vi "to_json.vi"(8 "error in":errorcluster, 11 "target.video in":refnum<class "target.video.lvclass">) -> (0 "error out":errorcluster, 2 "json":string, 3 "target.video out":refnum<class "target.video.lvclass">, 4 "Not Default":bool)   [LabVIEW 2020, in "datasources.lvlib" / "target.video.lvclass"]
uses:
  target.video.lvclass
  C:/code/labview-client/lv_src/Nominal Client/datasources/target/target.lvclass
  target.video.lvclass/target.video.ctl
  target/target.lvclass/target.ctl
  dataset/dataset.lvclass/dataset.ctl
  428e81a4-e553-4bd8-9727-470612eb2722.vi
  44014f50-ab4e-42bf-98e0-f8910821d057.vi
  6f4a9cd9-95da-4d00-8da6-4a49d3ace755.vi
  b2da3fc4-5a27-4170-9632-6c616410d1ce.vi
  a8577a1a-19ab-4315-acfd-5959197f0bba.vi
  b13016ed-5689-47b0-9406-ea70241d4c20.vi
  dd574b23-1e1f-49d0-b409-8656717e9e11.vi
  target/properties.get.vi
  target/labels.get.vi
  target/dataset.get.vi
  target/channelConfig.get.vi
  target/workspace.get.vi
  dataset/datasetName.get.vi
  dataset/datasetDescription.get.vi
  dataset/rid.get.vi
  <vilib>/JDP Science/JSONtext/Variant to JSON Text.vi
  <vilib>/JDP Science/JSONtext/support/Format JSON Object.vi
  nominal types/properties/properties.lvclass
  nominal types/labels/labels.lvclass
  <vilib>/JDP Science/JSONtext/LVClass Serializer/JSONtext LVClass Serializer.lvclass
  dataset/dataset.lvclass
  nominal types/channelConfig/channelConfig.lvclass
  nominal types/workspace/workspace.lvclass
  <vilib>/JDP Science/JSONtext/JSONtext.lvlib
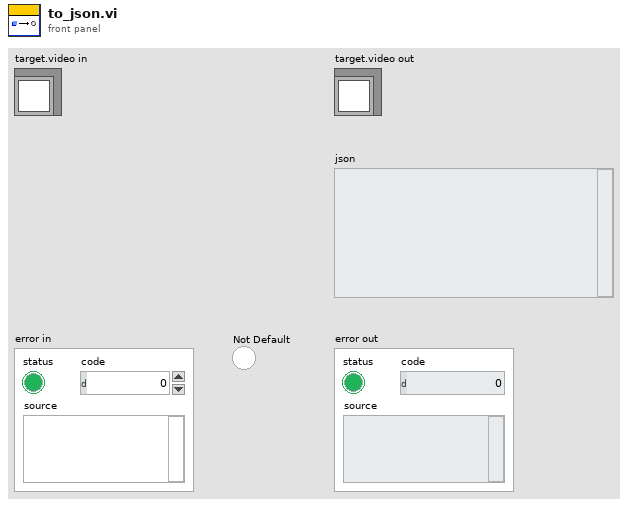
[diagram p1: front panel]
types:
  T1 = cluster{"type":string, "existing":cluster{"videoRid":string}}
  T2 = cluster{"Accessors:datasetName":string, "Accessors:datasetDescription":string}
  T3 = cluster{"Accessors:datasetName":bool, "Accessors:datasetDescription":bool}
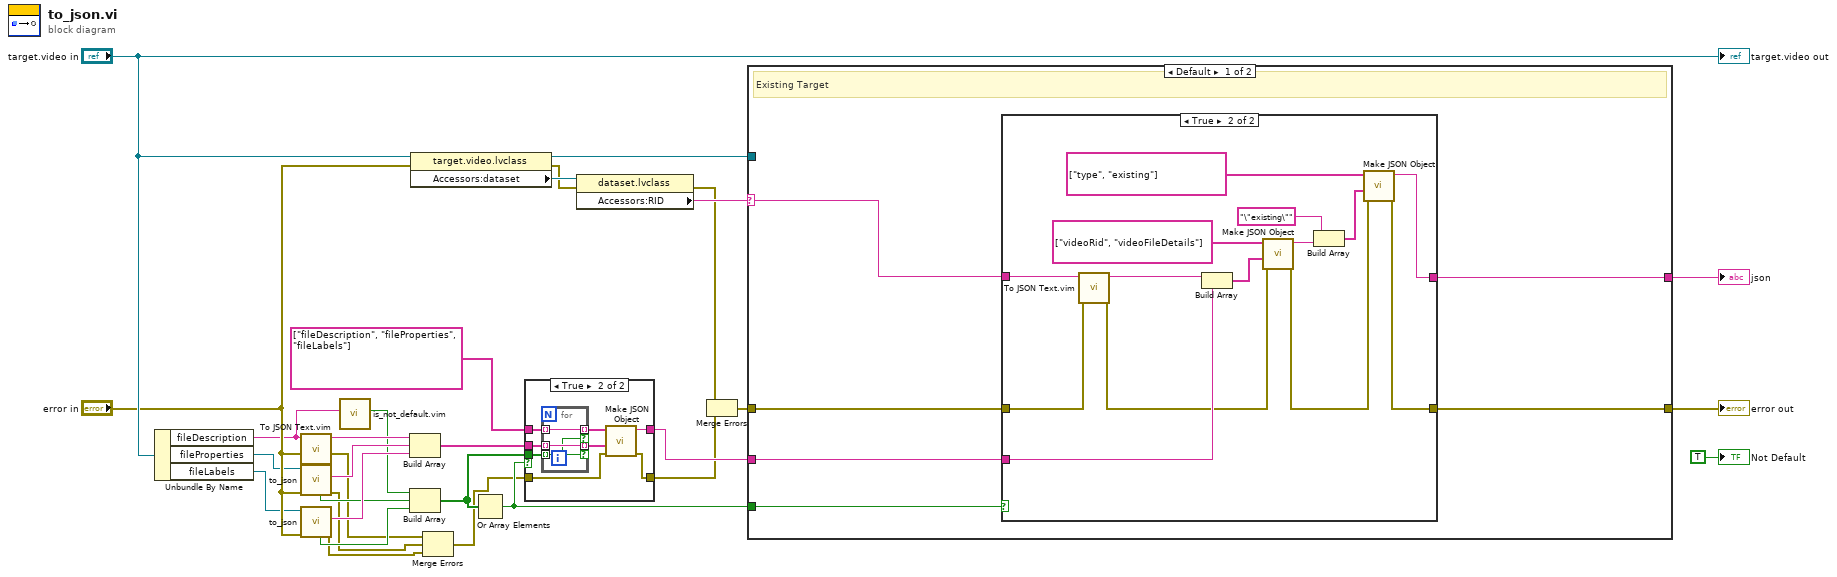
[diagram p0: block diagram]
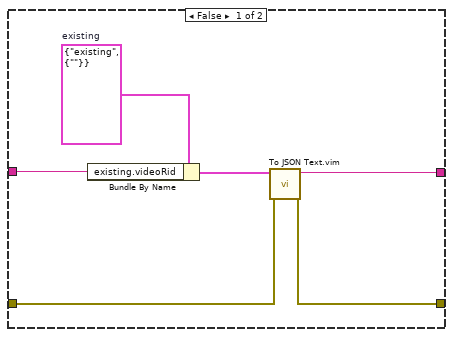
[diagram p3: hidden frame]
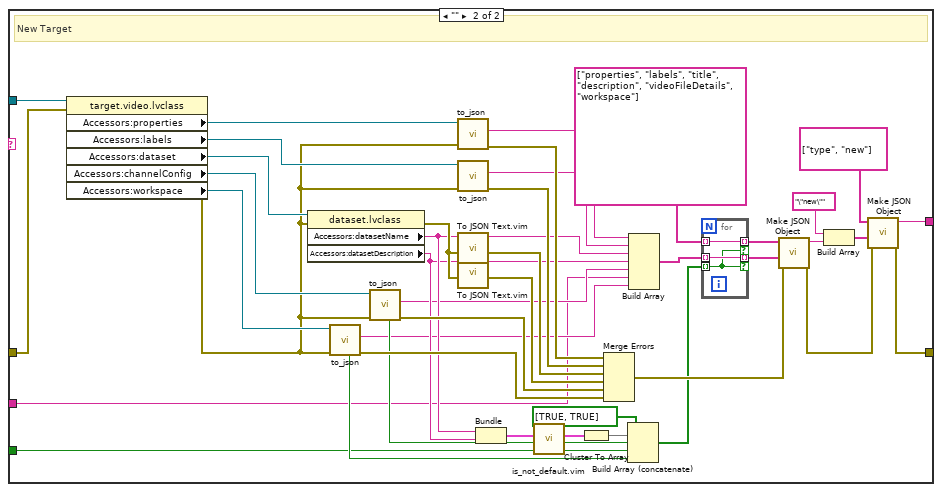
[diagram p4: hidden frame]
diagram:
  n1 = Unbundle By Name("target.video in") -> ("fileDescription"=w3:string, "fileProperties"=w2:refnum<class "properties.lvclass">, "fileLabels"=w1:refnum<class "labels.lvclass">)
  n2 = call "To JSON Text.vim"("error in (no error)"="error in", "Anything"=w3) -> ("error out"=w10:errorcluster, "<JSON>"=w20:string)  [unwired: 8 in]
  n3 = call-dynamic "to_json.vi"("error in"="error in", "properties in"=w2) -> ("error out"=w9:errorcluster, "json"=w22:string, "Not Default"=w18:bool)  [unwired: 6 in, 1 out]
  n4 = call-dynamic "to_json.vi"("error in"="error in", "labels in"=w1) -> ("error out"=w8:errorcluster, "json"=w21:string, "Not Default"=w19:bool)  [unwired: 6 in, 1 out]
  n5 = call "is_not_default.vim"("data"=w3) -> ("Not Default"=w17:bool)  [unwired: 10 in]
  n6 = Build Array(w20, w22, w21) -> (w23:string[])
  n7 = Build Array(w17, w18, w19) -> (w25:bool[])
  n8 = property class="target.video.lvclass"(reference="target.video in", error in="error in") -> (reference out=w13:refnum<class "target.video.lvclass">, error out=w11:errorcluster, "Accessors:dataset"=w29:refnum<class "dataset.lvclass">)
  n9 = Merge Errors(w10, w9, w8) -> (w7:errorcluster)
  n10 = Or Array Elements(Boolean array=w25) -> (logical OR=w14:bool)
  n11 = case shown="True" w14 {
    tunnel: w23 -> [_ w39]
    tunnel: string[] ["fileDescription", "fileProperties", "fileLabels"] ("Item Names") -> [_ w38]
    tunnel: w25 -> [_ w35]
    tunnel: [_ w34] -> w15
    tunnel: [w31 w33] -> w5
    tunnel: w7 -> [w31 w32]
    frame False {
    }
    frame True {
      n12 = for {
        tunnel: w39 -> [w42] mode=indexing
        tunnel: [w42] -> w36 mode=indexing if=w40
        tunnel: w38 -> [w41] mode=indexing
        tunnel: [w41] -> w37 mode=indexing if=w40
        tunnel: w35 -> [w40] mode=indexing
      }
      n13 = call <vilib>:"Make JSON Object.vi"("error in (no error)"=w32, "JSON Items"=w36, "Item Names"=w37) -> ("error out"=w33:errorcluster, "<JSON>"=w34:string)  [unwired: 7 in]
    }
  }
  n14 = property class="dataset.lvclass"(reference=w29, error in=w11) -> (error out=w6:errorcluster, "Accessors:RID"=w30:string)  [unwired: 1 out]
  n15 = Merge Errors(w6, w5) -> (w4:errorcluster)
  n16 = case shown="Default" w30 {
    selector: w30 -> [w48 _]
    tunnel: [w47 w96] -> w28
    tunnel: [w46 w94] -> w27
    tunnel: w15 -> [w43 w72]
    tunnel: w14 -> [w44 w70]
    tunnel: w13 -> [_ w71]
    tunnel: w4 -> [w45 w69]
    frame Default {
      # "Existing Target"
      n17 = case shown="True" w44 {
        tunnel: w48 -> [w53 w65]
        tunnel: [w51 w57] -> w47
        tunnel: [w50 w55] -> w46
        tunnel: w45 -> [w49 w63]
        tunnel: w43 -> [_ w67]
        frame False {
          w54 = T1 {"type"="existing", "existing"={"videoRid"=""}}  # existing
          n18 = Bundle By Name(cluster=w54, "existing.videoRid"=w53) -> (w52:T1)
          n19 = call "To JSON Text.vim"("error in (no error)"=w49, "Anything"=w52) -> ("error out"=w50:errorcluster, "<JSON>"=w51:string)  [unwired: 8 in]
        }
        frame True {
          n20 = call "To JSON Text.vim"("error in (no error)"=w63, "Anything"=w65) -> ("error out"=w62:errorcluster, "<JSON>"=w64:string)  [unwired: 8 in]
          n21 = Build Array(w64, w67) -> (w66:string[])
          n22 = call <vilib>:"Make JSON Object.vi"("error in (no error)"=w62, "JSON Items"=w66, "Item Names"=string[] ["videoRid", "videoFileDetails"]) -> ("error out"=w56:errorcluster, "<JSON>"=w59:string)  [unwired: 7 in]
          n23 = Build Array("\"existing\"", w59) -> (w58:string[])
          n24 = call <vilib>:"Make JSON Object.vi"("error in (no error)"=w56, "JSON Items"=w58, "Item Names"=string[] ["type", "existing"]) -> ("error out"=w55:errorcluster, "<JSON>"=w57:string)  [unwired: 7 in]
        }
      }
    }
    frame "" {
      # "New Target"
      n25 = property class="target.video.lvclass"(reference=w71, error in=w69) -> (error out=w75:errorcluster, "Accessors:properties"=w80:refnum<class "properties.lvclass">, "Accessors:labels"=w79:refnum<class "labels.lvclass">, "Accessors:dataset"=w78:refnum<class "dataset.lvclass">, "Accessors:channelConfig"=w77:refnum<class "channelConfig.lvclass">, "Accessors:workspace"=w76:refnum<class "workspace.lvclass">)  [unwired: 1 out]
      n26 = property class="dataset.lvclass"(reference=w78, error in=w75) -> (error out=w112:errorcluster, "Accessors:datasetName"=w84:string, "Accessors:datasetDescription"=w83:string)  [unwired: 1 out]
      n27 = call-dynamic "to_json.vi"("error in"=w75, "workspace in"=w76) -> ("error out"=w102:errorcluster, "json"=w74:string, "Not Default"=w73:bool)  [unwired: 6 in, 1 out]
      n28 = call-dynamic "to_json.vi"("error in"=w75, "channelConfig in"=w77) -> ("error out"=w107:errorcluster, "json"=w82:string, "Not Default"=w81:bool)  [unwired: 6 in, 1 out]
      n29 = call-dynamic "to_json.vi"("error in"=w75, "properties in"=w80) -> ("error out"=w111:errorcluster, "json"=w106:string)  [unwired: 6 in, 2 out]
      n30 = call-dynamic "to_json.vi"("error in"=w75, "labels in"=w79) -> ("error out"=w110:errorcluster, "json"=w105:string)  [unwired: 6 in, 2 out]
      n31 = call "To JSON Text.vim"("error in (no error)"=w112, "Anything"=w84) -> ("error out"=w109:errorcluster, "<JSON>"=w104:string)  [unwired: 8 in]
      n32 = call "To JSON Text.vim"("error in (no error)"=w112, "Anything"=w83) -> ("error out"=w108:errorcluster, "<JSON>"=w103:string)  [unwired: 8 in]
      n33 = Bundle("Accessors:datasetName"=w84, "Accessors:datasetDescription"=w83) -> (w89:T2)  [unwired: 1 in]
      n34 = call "is_not_default.vim"("data"=w89) -> ("Not Default"=w88:T3)  [unwired: 10 in]
      n35 = Cluster To Array(cluster=w88) -> (array=w87:bool[])
      n36 = Merge Errors(w111, w110, w109, w108, w107, w102) -> (w101:errorcluster)
      n37 = Build Array (concatenate)(bool[] [TRUE, TRUE] ("element"), w87, w81, w70, w73) -> (w85:bool[])
      n38 = Build Array(w106, w105, w104, w103, w82, w72, w74) -> (w93:string[])
      n39 = for {
        tunnel: w93 -> [w115] mode=indexing
        tunnel: [w115] -> w92 mode=indexing if=w113
        tunnel: string[] ["properties", "labels", "title", "description", "videoFileDetails", "workspace"] ("Item Names") -> [w114] mode=indexing
        tunnel: [w114] -> w90 mode=indexing if=w113
        tunnel: w85 -> [w113] mode=indexing
      }
      n40 = call <vilib>:"Make JSON Object.vi"("error in (no error)"=w101, "JSON Items"=w92, "Item Names"=w90) -> ("error out"=w95:errorcluster, "<JSON>"=w99:string)  [unwired: 7 in]
      n41 = Build Array("\"new\"" ("element"), w99) -> (w97:string[])
      n42 = call <vilib>:"Make JSON Object.vi"("error in (no error)"=w95, "JSON Items"=w97, "Item Names"=string[] ["type", "new"]) -> ("error out"=w94:errorcluster, "<JSON>"=w96:string)  [unwired: 7 in]
    }
  }
  "error out" <- w27
  "json" <- w28
  "target.video out" <- "target.video in"
  "Not Default" <- TRUE ("Not Default")
